vi "Update Pattern.vi"(8 "error in (no error)":errorcluster, 11 "Grid Animation in":refnum<class "Grid Animation.lvclass">) -> (0 "error out":errorcluster, 3 "Grid Animation out":refnum<class "Grid Animation.lvclass">)   [LabVIEW 2021, in "Grid Animation.lvlib" / "Grid Animation.lvclass"]
uses:
  Grid Animation.lvclass
  Grid Animation.lvclass/Grid Animation.ctl
  MC Screen/Grid Screen Messages/Set Grid Value Using Coordinates Msg/Set Grid Value Using Coordinates Msg.lvclass/Set Grid Value Using Coordinates Msg.ctl
  <vilib>/ActorFramework/Message Enqueuer/Message Enqueuer.lvclass/Message Enqueuer.ctl
  <vilib>/ActorFramework/Message Enqueuer/Enqueue.vi
  MC Screen/Grid Screen Messages/Set Grid Value Using Coordinates Msg/Set Grid Value Using Coordinates Msg.lvclass
  C:/Program Files/National Instruments/LabVIEW 2024/vi.lib/ActorFramework/Message/Message.lvclass
  <vilib>/ActorFramework/Message Priority Queue/Priority Enqueue.vi
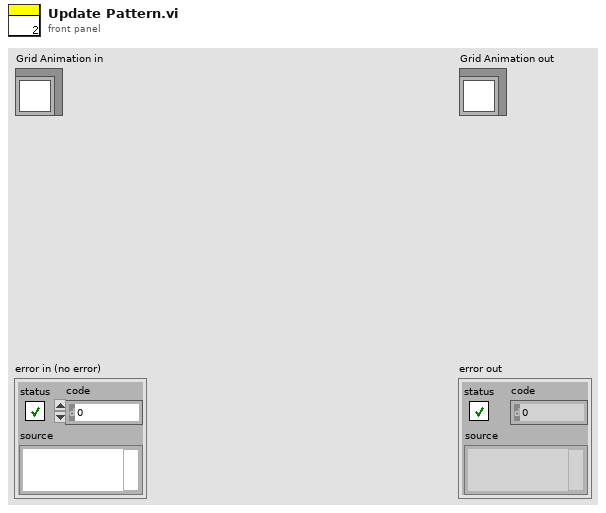
[diagram p1: front panel]
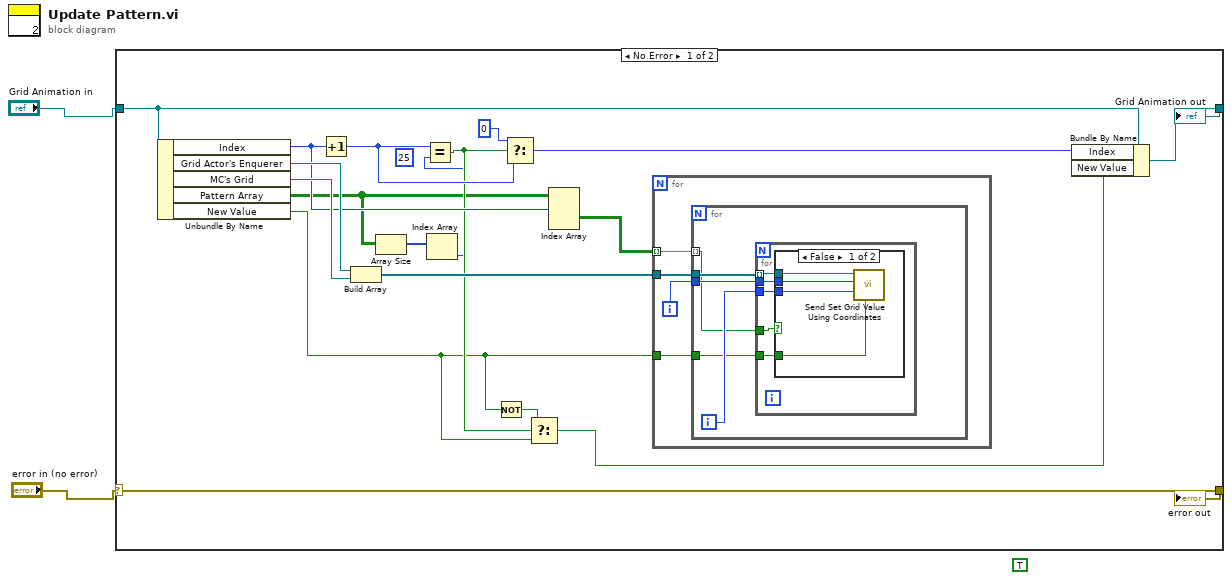
[diagram p0: block diagram]
diagram:
  (unwired) TRUE
  n1 = case shown="No Error" "error in (no error)" {
    selector: "error in (no error)" -> [w22 w42]
    tunnel: [w22 w42] -> w3
    tunnel: [w21 w41] -> w1
    tunnel: "Grid Animation in" -> [w20 w41]
    frame No Error {
      (unwired) 25 ("y")
      n2 = Unbundle By Name(w20) -> ("Index"=w12:i32, "Grid Actor's Enquerer"=w17:refnum<class "Message Enqueuer.lvclass">, "MC's Grid"=w16:refnum<class "Message Enqueuer.lvclass">, "Pattern Array"=w7:bool[][][], "New Value"=w9:bool)
      n3 = Increment(x=w12) -> (x+1=w13:i32)
      n4 = Build Array(w17, w16) -> (w15:refnum<class "Message Enqueuer.lvclass">[])
      n5 = Array Size(array=w7) -> (size(s)=w6:i32[])
      n6 = Index Array(array=w6) -> (element=w5:i32)  [unwired: 1 in]
      n7 = Equal?(x=w13, y=w5) -> (x = y?=w11:bool)
      n8 = Not(x=w9) -> (.not. x?=w10:bool)
      n9 = Select(t=0, s=w11, f=w13) -> (s? t:f=w18:i32)
      n10 = Select(t=w10, s=w11, f=w9) -> (s? t:f=w8:bool)
      n11 = Index Array(array=w7, index (dim 0)=w12) -> (element=w14:bool[][])  [unwired: 2 in]
      n12 = for {
        tunnel: w15 -> [w26]
        tunnel: w14 -> [w25] mode=indexing
        tunnel: w9 -> [w23]
        i -> [w24]
        n13 = for {
          tunnel: w26 -> [w31]
          tunnel: w25 -> [w28] mode=indexing
          tunnel: w24 -> [w30]
          tunnel: w23 -> [w27]
          i -> [w29]
          n14 = for {
            tunnel: w31 -> [w36] mode=indexing
            tunnel: w30 -> [w35]
            tunnel: w29 -> [w34]
            tunnel: w28 -> [w33]
            tunnel: w27 -> [w32]
            n15 = case shown="False" w33 {
              tunnel: w36 -> [w40 _]
              tunnel: w35 -> [w39 _]
              tunnel: w34 -> [w38 _]
              tunnel: w32 -> [w37 _]
              frame False {
                n16 = call "Send Set Grid Value Using Coordinates.vi"("Cell Value"=w37, "Row"=w38, "Column"=w39, "Message Enqueuer"=w40) -> ()  [unwired: 6 in, 2 out]
              }
              frame True {
              }
            }
          }
        }
      }
      n17 = Bundle By Name(cluster=w20, "Index"=w18, "New Value"=w8) -> (w21:refnum<class "Grid Animation.lvclass">)
    }
    frame Error {
    }
  }
  "error out" <- w3
  "Grid Animation out" <- w1
